vi "MCS_StopAction.vi"(1 "error in (no error)":errorcluster, 2 "Channel Index In":u32, 3 "System Index In":u32) -> (0 "error out":errorcluster)   [LabVIEW 2010]
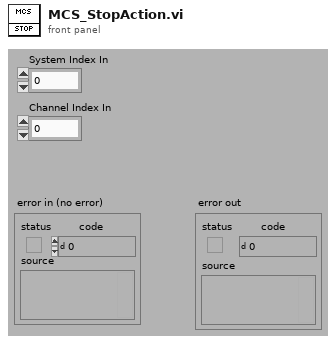
[diagram p1: front panel]
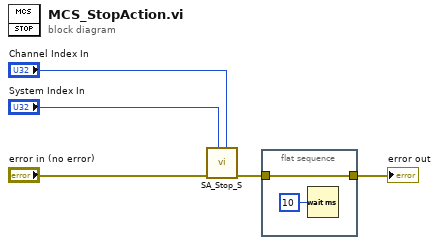
[diagram p0: block diagram]
diagram:
  n1 = call <vilib>:"SA_Stop_S.vi"("channelIndex"="Channel Index In", "systemIndex"="System Index In", "error in (no error)"="error in (no error)") -> ("error out"=w2:errorcluster)  [unwired: 8 in]
  n2 = flat-sequence {
    tunnel: w2 -> [w6]
    tunnel: [w6] -> w1
    frame #0 {
      n3 = Wait (ms)(milliseconds to wait=u32 10) -> ()  [unwired: 1 out]
    }
  }
  "error out" <- w1
